vi "Use Adaptive Filter (Waveform).vi"() -> ()   [LabVIEW 2019]
doc: "This example demonstrates how to create and use an adaptive filter. This example simulates and filters signals as waveforms.\n\nComplete the following steps to use this example.\n\n1. Run this VI. Observe how the coefficients of the adaptive filter converge to those of the unknown system.\n\n2. Browse the block diagram of this example to understand how this example uses the adaptive filter VIs.\n\n3. Replace the AFT Create FIR LMS VI with other filter creation VIs palette to try other adaptive filter algorithms.\n\nThis example uses an FIR LMS adaptive filter to identify the impulse response of an unknown system. A lowpass FIR filter simulates the unknown system. The input to both this system and the adaptive filter is Gaussian white noise. The output of this system is the reference of the adaptive filter."
uses:
  <vilib>/addons/Adaptive Filters/Create/AFT Create FIR LMS (Real).vi
  <vilib>/addons/Adaptive Filters/Processing/AFT Filter Signal and Update Coefficients (Real, Waveform).vi
  <vilib>/addons/Adaptive Filters/Analysis/AFT Get Coefficients (FIR, Real).vi
  <vilib>/addons/Adaptive Filters/NI_AdaptiveFilter.lvlib
panel:
  in  "Stop":bool
  out "Error Signal":waveform(dbl)(graph)
  in  "Step Size":dbl=0.002 min=0.0 step=0.001
  in  "Filter Length":i32=25 min=2
  out "Coefficients":dbl[][](graph)
  # "Select Help>>Show Context Help and move the cursor over the VI icon of this example for more information."
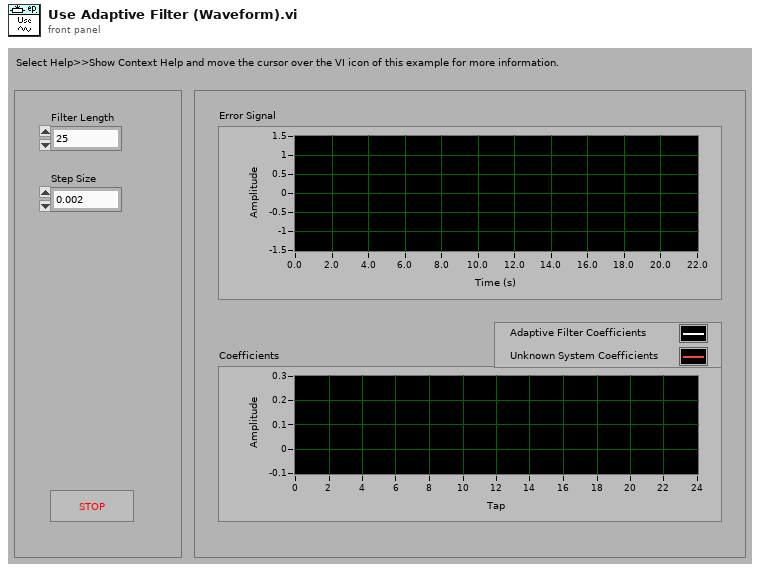
[diagram p1: front panel]
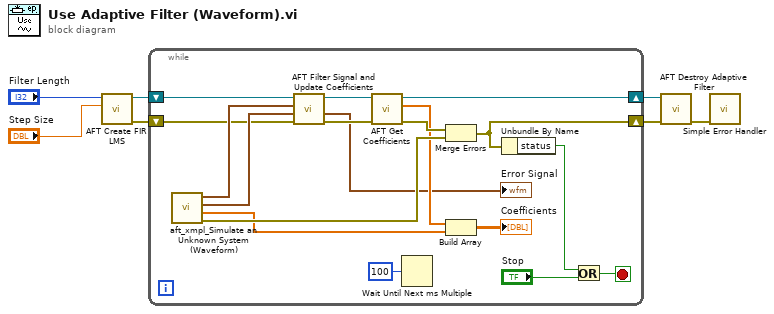
[diagram p0: block diagram]
diagram:
  n1 = call-poly <vilib>:"AFT Create FIR LMS.vi"("step size"="Step Size", "filter length"="Filter Length") -> ("error out"=w4:errorcluster, "adaptive filter out"=w6:refnum<k20>)  [unwired: 2 in, 6 out]
  n2 = while {
    shift-right: [w13] -> w2
    shift-left: w6 -> [w23]
    shift-right: [w8] -> w3
    shift-left: w4 -> [w15]
    stop <- w10 stop-if-true
    n3 = call "aft_xmpl_Simulate an Unknown System (Waveform).vi"() -> ("error out"=w24:errorcluster, "unknown system coefficients"=w14:dbl[], "response signal"=w17:waveform(dbl), "stimulus signal"=w18:waveform(dbl))  [unwired: 4 in, 4 out]
    n4 = call-poly <vilib>:"AFT Filter Signal and Update Coefficients.vi"("error in (no error)"=w15, "d(n)"=w17, "x(n)"=w18, "adaptive filter in"=w23) -> ("error out"=w21:errorcluster, "e(n)"=→"Error Signal":waveform(dbl), "adaptive filter out"=w22:refnum<k20>)  [unwired: 2 in, 3 out]
    n5 = call-poly <vilib>:"AFT Get Coefficients.vi"("error in (no error)"=w21, "adaptive filter in"=w22) -> ("error out"=w25:errorcluster, "coefficients"=w20:dbl[], "adaptive filter out"=w13:refnum<k20>)  [unwired: 7 out]
    n6 = Wait Until Next ms Multiple(millisecond multiple=u32 100) -> ()  [unwired: 1 out]
    n7 = Merge Errors(w25, w24) -> (w8:errorcluster)
    n8 = Build Array(w20, w14) -> (→"Coefficients":dbl[][])
    n9 = Unbundle By Name(w8) -> ("status"=w12:bool)
    n10 = Or(x=w12, y="Stop") -> (x .or. y?=w10:bool)
  }
  n11 = call <vilib>:"AFT Destroy Adaptive Filter.vi"("error in (no error)"=w3, "adaptive filter in"=w2) -> ("error out"=w1:errorcluster)  [unwired: 9 out]
  n12 = call <vilib>:"Simple Error Handler.vi"("error in (no error)"=w1) -> ()  [unwired: 1 in, 8 out]
